vi "Pixel 5 Condition (SubVI).vi"(8 "Image Width":u16=240, 10 "Contour Scan in":T1, 11 "Fnd?":bool) -> (2 "Contour Scan out":T1)   [LabVIEW 2015]
uses:
  Controls (FPGA)/Contour Scan.ctl
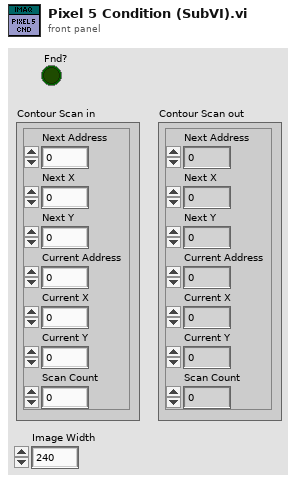
[diagram p1: front panel]
types:
  T1 = typedef "Contour Scan.ctl" = cluster{"Next Address":fxp<+,24,24>, "Next X":fxp<+,12,12>, "Next Y":fxp<+,12,12>, "Current Address":fxp<+,24,24>, "Current X":fxp<+,12,12>, "Current Y":fxp<+,12,12>, "Scan Count":u32}
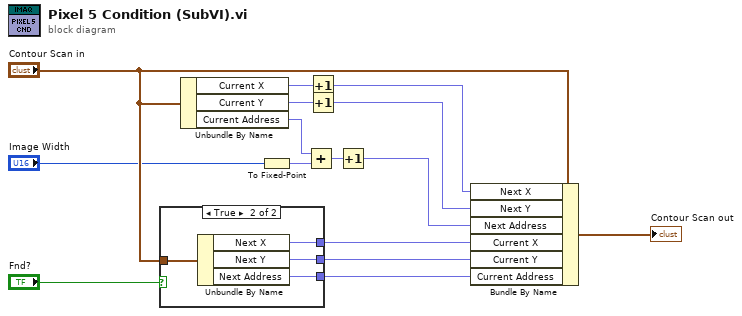
[diagram p0: block diagram]
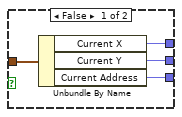
[diagram p2: hidden frame]
diagram:
  n1 = case shown="True" "Fnd?" {
    tunnel: "Contour Scan in" -> [w19 w23]
    tunnel: [w18 w22] -> w13
    tunnel: [w17 w21] -> w14
    tunnel: [w16 w20] -> w15
    frame False {
      n2 = Unbundle By Name(w19) -> ("Current X"=w18:fxp<+,12,12>, "Current Y"=w17:fxp<+,12,12>, "Current Address"=w16:fxp<+,24,24>)
    }
    frame True {
      n3 = Unbundle By Name(w23) -> ("Next X"=w22:fxp<+,12,12>, "Next Y"=w21:fxp<+,12,12>, "Next Address"=w20:fxp<+,24,24>)
    }
  }
  n4 = Unbundle By Name("Contour Scan in") -> ("Current X"=w10:fxp<+,12,12>, "Current Y"=w8:fxp<+,12,12>, "Current Address"=w4:fxp<+,24,24>)
  n5 = To Fixed-Point(number="Image Width") -> (fixed-point=w6:fxp<+,12,12>)  [unwired: 1 in]
  n6 = Add(x=w4, y=w6) -> (x+y=w5:fxp<+,24,24>)
  n7 = Increment(x=w10) -> (x+1=w3:fxp<+,12,12>)
  n8 = Increment(x=w8) -> (x+1=w7:fxp<+,12,12>)
  n9 = Increment(x=w5) -> (x+1=w2:fxp<+,24,24>)
  n10 = Bundle By Name(cluster="Contour Scan in", "Next X"=w3, "Next Y"=w7, "Next Address"=w2, "Current X"=w13, "Current Y"=w14, "Current Address"=w15) -> (→"Contour Scan out":T1)
